vi "Echo.vi"(8 "error in (no error)":errorcluster, 10 "Error In":errorcluster, 11 "Level1Handler in":refnum<class "Level1Handler.lvclass">) -> (0 "error out":errorcluster, 1 "Still Pass?":bool, 2 "handled?":bool, 3 "Level1Handler out":refnum<class "Level1Handler.lvclass">)   [LabVIEW 2014, in "Chain Of Responsibility Pattern.lvlib" / "Level1Handler.lvclass"]
uses:
  Level1Handler.lvclass
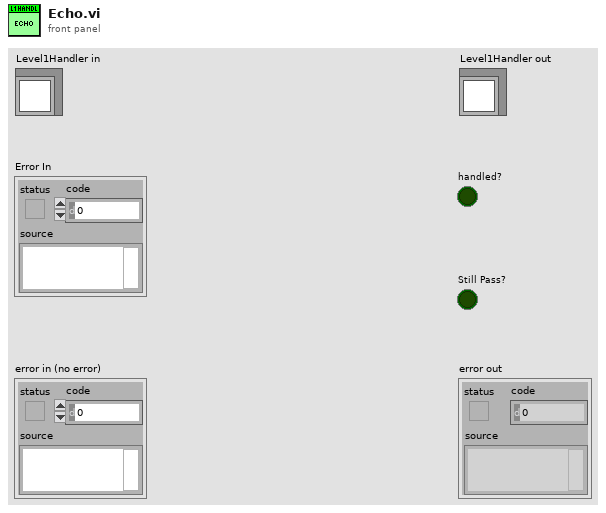
[diagram p1: front panel]
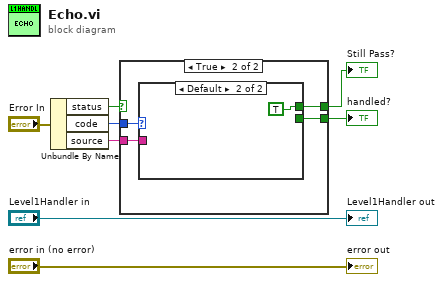
[diagram p0: block diagram]
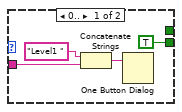
[diagram p3: hidden frame]
diagram:
  n1 = Unbundle By Name("Error In") -> ("status"=w2:bool, "code"=w7:i32, "source"=w5:string)
  n2 = case shown="True" w2 {
    tunnel: w7 -> [_ w12]
    tunnel: [_ w11] -> w6
    tunnel: w5 -> [_ w10]
    tunnel: [_ w9] -> w4
    frame False {
    }
    frame True {
      n3 = case shown="Default" w12 {
        tunnel: [_ TRUE] -> w11
        tunnel: w10 -> [w16 _]
        tunnel: [TRUE _] -> w9
        frame 0.. {
          n4 = Concatenate Strings("Level1 " ("string"), w16) -> (w15:string)
          n5 = One Button Dialog(message=w15) -> ()  [unwired: 1 in, 1 out]
        }
        frame Default {
        }
      }
    }
  }
  "Still Pass?" <- w6
  "handled?" <- w4
  "error out" <- "error in (no error)"
  "Level1Handler out" <- "Level1Handler in"
